vi "PPS Delimited string to boolean array.vi"(10 "delimiter":string="\t", 11 "1D string of Booleans separated by delimiter":string="1\t2\t3\t4\t") -> (3 "Boolean array":bool[](array[boolean]))   [LabVIEW 2016]
uses:
  <vilib>/Utility/error.llb/whitespace.ctl
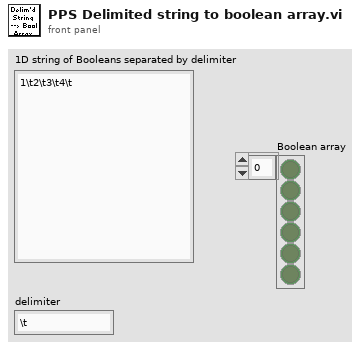
[diagram p1: front panel]
types:
  T1 = typedef "whitespace.ctl" = u16
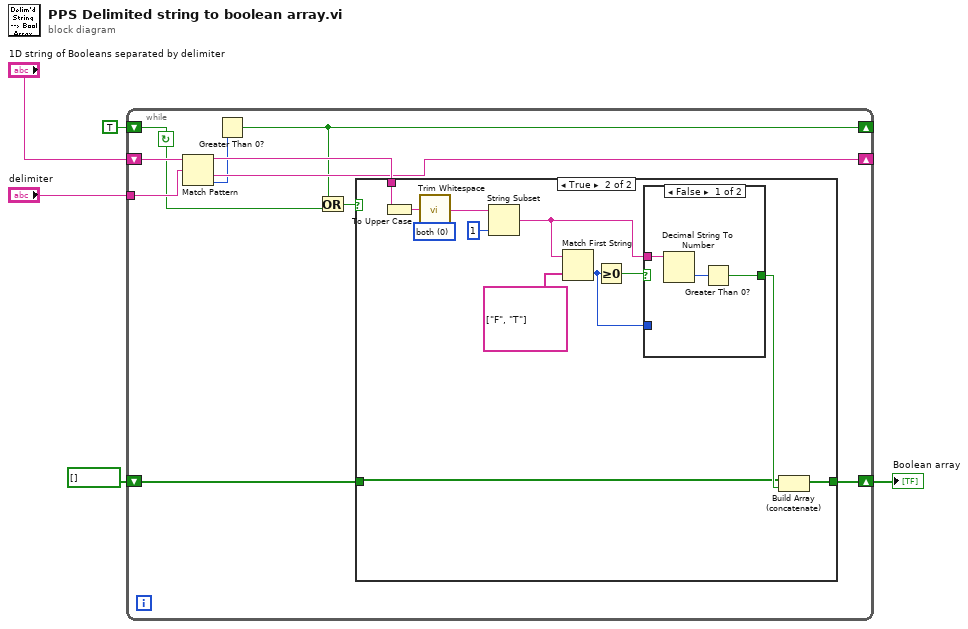
[diagram p0: block diagram]
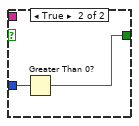
[diagram p3: hidden frame]
diagram:
  n1 = while {
    shift-right: [w10] -> _
    shift-left: "1D string of Booleans separated by delimiter" -> [w15]
    shift-right: [w12] -> w3
    shift-left: bool[] [] -> [w13]
    tunnel: "delimiter" -> [w11]
    shift-right: [w8] -> _
    shift-left: TRUE -> [w7]
    stop <- w7 continue-if-true
    n2 = Match Pattern(string=w15, regular expression=w11) -> (before substring=w14:string, after substring=w10:string, offset past match=w9:i32)  [unwired: 1 in, 1 out]
    n3 = Greater Than 0?(x=w9) -> (x > 0?=w8:bool)
    n4 = Or(x=w8, y=w7) -> (x .or. y?=w6:bool)
    n5 = case shown="True" w6 {
      tunnel: w14 -> [_ w28]
      tunnel: w13 -> [w16 w17]
      tunnel: [w16 w18] -> w12
      frame False {
      }
      frame True {
        w25 = T1 0 items=["both", "start of string", "end of string"] ("location (both)")
        n6 = To Upper Case(1:w28) -> (0:w26:string)
        n7 = call <vilib>:"Trim Whitespace.vi"("string"=w26, "location (both)"=w25) -> ("trimmed string"=w24:string)
        n8 = String Subset(string=w24, length (rest)=1 ("length (rest)")) -> (substring=w20:string)  [unwired: 1 in]
        n9 = Match First String(2:string[] ["F", "T"] ("string array"), 3:w20) -> (0:w21:i32)  [unwired: 1 out]
        n10 = Greater Or Equal To 0?(x=w21) -> (x >= 0?=w22:bool)
        n11 = case shown="False" w22 {
          tunnel: w21 -> [_ w33]
          tunnel: w20 -> [w30 _]
          tunnel: [w29 w32] -> w19
          frame False {
            n12 = Decimal String To Number(string=w30) -> (number=w31:i32)  [unwired: 2 in, 1 out]
            n13 = Greater Than 0?(x=w31) -> (x > 0?=w29:bool)
          }
          frame True {
            n14 = Greater Than 0?(x=w33) -> (x > 0?=w32:bool)
          }
        }
        n15 = Build Array (concatenate)(w17, w19) -> (w18:bool[])
      }
    }
  }
  "Boolean array" <- w3
